vi "WPI_CameraGet Exposure Priority.vi"(8 "error in (no error)":errorcluster, 11 "CameraDevRef":T1={"Camera Address"="192.168.0.90", "CameraStatus"={"status"=FALSE, "code"=0, "source"=""}}) -> (0 "error out":errorcluster, 2 "Exposure Priority":T2, 3 "CameraDevRef Out":T1)   [LabVIEW 2017]
doc: "Returns whether the camera you specify prioritizes the frame rate or image quality when setting the exposure.\n\nThis software is licensed. Open the labview\\readme\\WPI Robotics Library Open Source License.txt file for more information."
uses:
  <vilib>/Rock Robotics/WPI/Camera/WPI_CameraExposure Priority Values.ctl
  <vilib>/Rock Robotics/WPI/Camera/WPI_CameraDevRef.ctl
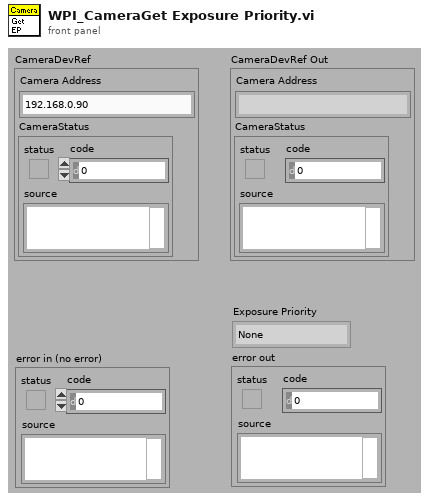
[diagram p1: front panel]
types:
  T1 = typedef "WPI_CameraDevRef.ctl" = cluster{"Camera Address":string, "CameraStatus":errorcluster}
  T2 = typedef "WPI_CameraExposure Priority Values.ctl" = enum16{"None", "Prioritize frame rate", "Prioritize image quality"}
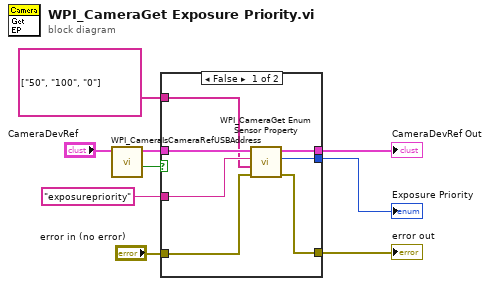
[diagram p0: block diagram]
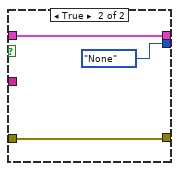
[diagram p2: hidden frame]
diagram:
  n1 = call <vilib>:"WPI_CameraIsCameraRefUSBAddress.vi"("CameraDevRef"="CameraDevRef") -> ("USB?"=w4:bool, "CameraDevRef out"=w2:T1)  [unwired: 7 in, 2 out]
  n2 = case shown="False" w4 {
    tunnel: "exposurepriority" ("format string") -> [w16 _]
    tunnel: "error in (no error)" -> [w15 w17]
    tunnel: [w14 WPI_CameraExposure_Priority_Values."None" ("Exposure Priority")] -> w7
    tunnel: [w13 w19] -> w6
    tunnel: [w12 w17] -> w5
    tunnel: w2 -> [w11 w19]
    tunnel: string[] ["50", "100", "0"] -> [w10 _]
    frame False {
      n3 = call <vilib>:"WPI_CameraGet Enum Sensor Property.vi"("error in (no error)"=w15, "Strings"=w10, "Property Name"=w16, "CameraDevRef"=w11) -> ("error out"=w12:errorcluster, "Enum Int Value"=w14:i32, "CameraDevRef out"=w13:T1)  [unwired: 2 in, 3 out]
    }
    frame True {
    }
  }
  "Exposure Priority" <- w7
  "CameraDevRef Out" <- w6
  "error out" <- w5
